vi "ENPID.vi"(2 "PID Settings":T1={"Gains"={"K(e)"=0.0, "Kp"=0.800000011920929, "Ki"=0.0, "Kd"=0.003000000026077032}, "Non-linear gain"={"Non-linear gain P"=enum."off", "Non-linear gain I"=enum."off", "Non-linear gain D"=enum."off"}, "D-Part variable"=enum."process variable", "Velocity estimate dy/dt"=enum."external", "Anti reset windup"=TRUE, "I-Part error band"=inf, "Output range"={"output high"=0.0, "output low"=0.0}}, 7 "r":dbl, 8 "Reset?":bool, 9 "y":dbl, 11 "dy/dt":dbl, 13 "dt (s)":dbl) -> (15 "u":dbl, 18 "u":cluster{"up":dbl, "ui":dbl, "ud":dbl, "u":dbl})   [LabVIEW 2019]
uses:
  PID_Settings.ctl
  Gains.ctl
  NonLinearGainParams.ctl
  NonLinearGain.ctl
  DPartVariable.ctl
  VelocityEstimate.ctl
  OutputRange.ctl
panel:
  # "Params"
  # "Input"
  # "Output"
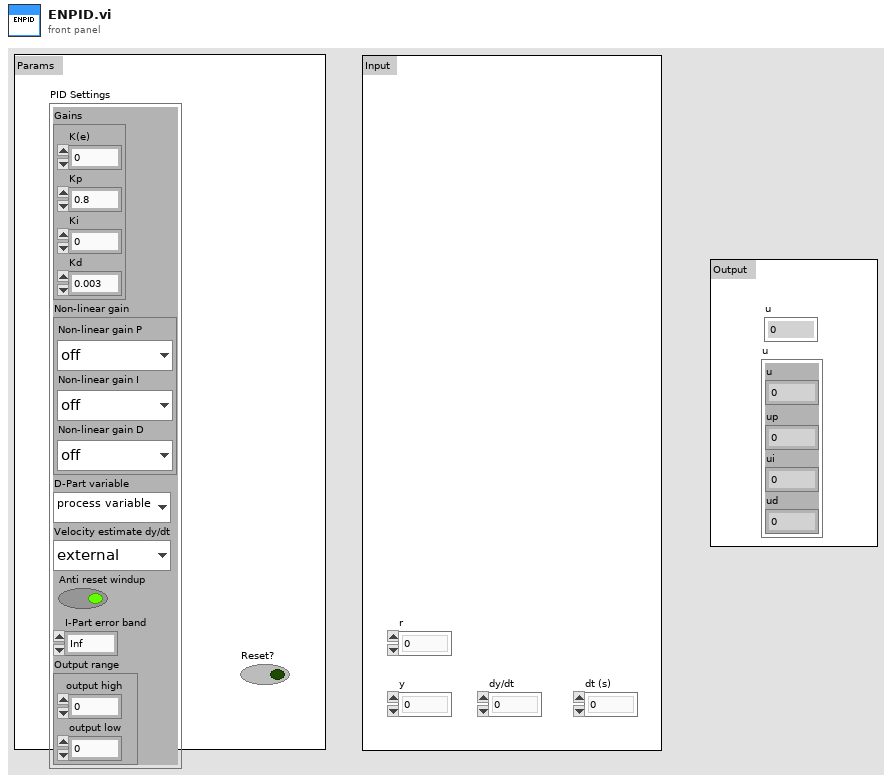
[diagram p1: front panel]
types:
  T1 = typedef "PID_Settings.ctl" = cluster{"Gains":T2, "Non-linear gain":T3, "D-Part variable":T5, "Velocity estimate dy/dt":T6, "Anti reset windup":bool, "I-Part error band":dbl, "Output range":T7}
  T2 = typedef "Gains.ctl" = cluster{"K(e)":dbl, "Kp":dbl, "Ki":dbl, "Kd":dbl}
  T3 = typedef "NonLinearGainParams.ctl" = cluster{"Non-linear gain P":T4, "Non-linear gain I":T4, "Non-linear gain D":T4}
  T4 = typedef "NonLinearGain.ctl" = enum16{"exponential", "quadratic", "off"}
  T5 = typedef "DPartVariable.ctl" = enum16{"error", "process variable"}
  T6 = typedef "VelocityEstimate.ctl" = enum16{"derivative", "external"}
  T7 = typedef "OutputRange.ctl" = cluster{"output high":dbl, "output low":dbl}
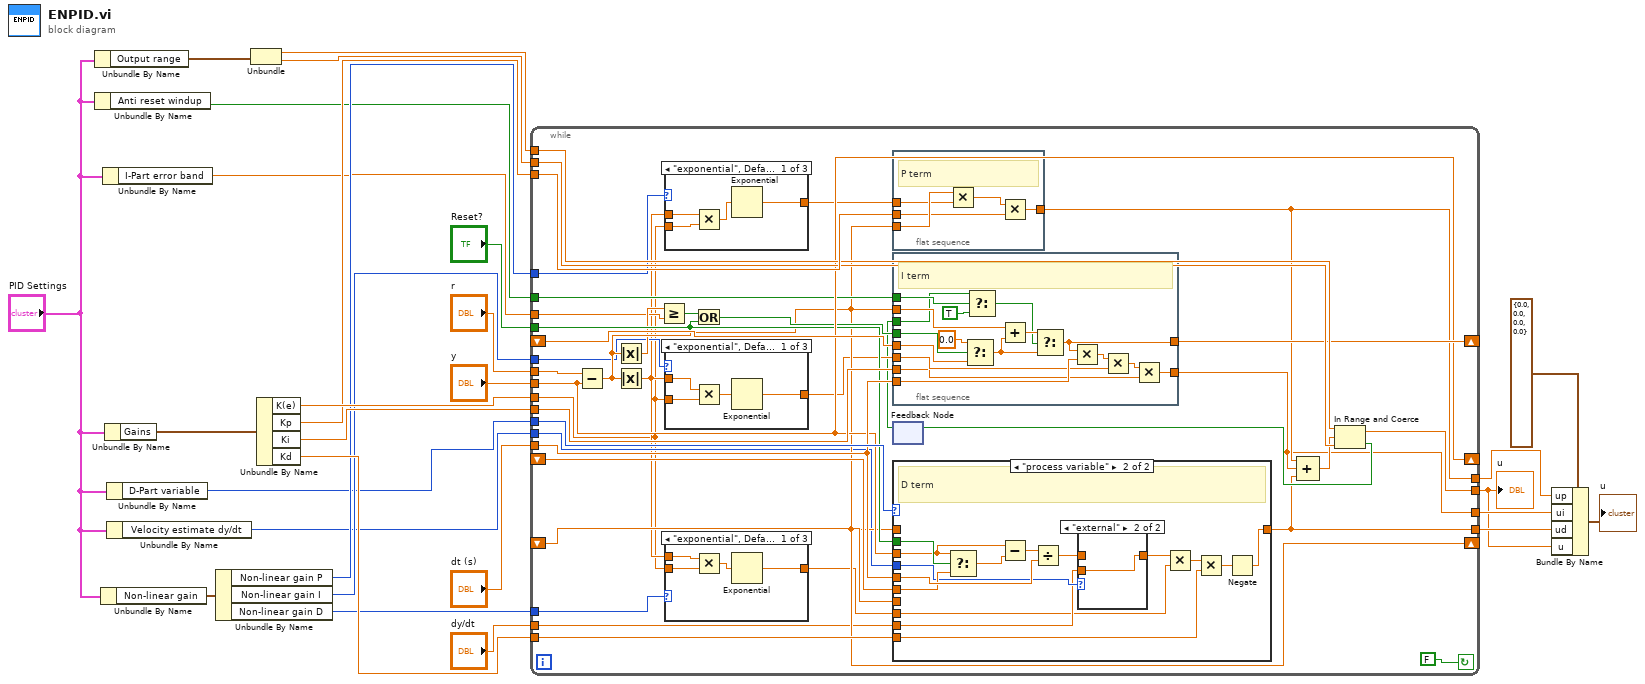
[diagram p0: block diagram]
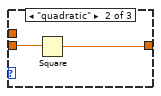
[diagram p2: hidden frame]
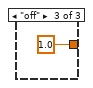
[diagram p3: hidden frame]
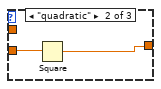
[diagram p4: hidden frame]
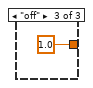
[diagram p5: hidden frame]
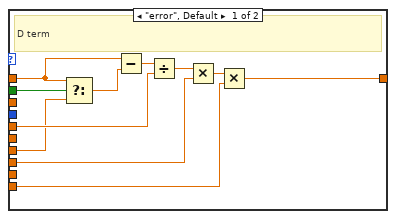
[diagram p6: hidden frame]
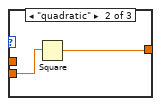
[diagram p8: hidden frame]
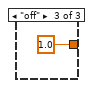
[diagram p9: hidden frame]
diagram:
  n1 = Unbundle By Name("PID Settings") -> ("Output range"=w2:T7)
  n2 = Unbundle By Name("PID Settings") -> ("Anti reset windup"=w7:bool)
  n3 = Unbundle By Name("PID Settings") -> ("Non-linear gain"=w8:T3)
  n4 = Unbundle By Name("PID Settings") -> ("I-Part error band"=w6:dbl)
  n5 = Unbundle By Name("PID Settings") -> ("Gains"=w9:T2)
  n6 = Unbundle By Name("PID Settings") -> ("D-Part variable"=w5:T5)
  n7 = Unbundle By Name("PID Settings") -> ("Velocity estimate dy/dt"=w4:T6)
  n8 = Unbundle By Name(w8) -> ("Non-linear gain P"=w10:T4, "Non-linear gain I"=w12:T4, "Non-linear gain D"=w11:T4)
  n9 = Unbundle(w2) -> ("output high"=w23:dbl, "output low"=w24:dbl)
  n10 = Unbundle By Name(w9) -> ("K(e)"=w28:dbl, "Kp"=w25:dbl, "Ki"=w20:dbl, "Kd"=w19:dbl)
  n11 = while {
    tunnel: w28 -> [w35]
    tunnel: "r" -> [w66]
    tunnel: "y" -> [w53]
    tunnel: w25 -> [w65]
    shift-right: [w42] -> _
    shift-left: _ -> [w50]
    tunnel: [w63] -> w1
    tunnel: w24 -> [w62]
    tunnel: w23 -> [w61]
    tunnel: "Reset?" -> [w45]
    tunnel: "dt (s)" -> [w55]
    tunnel: w20 -> [w56]
    shift-right: [w59] -> _
    shift-left: _ -> [w58]
    tunnel: w5 -> [w57]
    tunnel: w19 -> [w54]
    shift-right: [w53] -> _
    shift-left: _ -> [w52]
    tunnel: [w49] -> w18
    tunnel: [w48] -> w17
    tunnel: [w47] -> w16
    tunnel: w7 -> [w46]
    tunnel: w6 -> [w40]
    tunnel: "dy/dt" -> [w39]
    tunnel: w4 -> [w38]
    tunnel: w12 -> [w37]
    tunnel: w11 -> [w34]
    tunnel: w10 -> [w33]
    stop <- FALSE continue-if-true
    n12 = Subtract(x=w66, y=w53) -> (x-y=w42:dbl)
    n13 = Absolute Value(x=w42) -> (abs(x)=w41:dbl)
    n14 = Absolute Value(x=w42) -> (abs(x)=w36:dbl)
    n15 = Greater Or Equal?(x=w41, y=w40) -> (x >= y?=w43:bool)
    n16 = case shown="\"exponential\", Default" w33 {
      tunnel: w35 -> [w132 w136 _]
      tunnel: [w134 w135 1.0] -> w32
      tunnel: w36 -> [w131 _ _]
      frame "exponential", Default {
        n17 = Multiply(x=w131, y=w132) -> (x*y=w133:dbl)
        n18 = Exponential(1:w133) -> (0:w134:dbl)
      }
      frame "quadratic" {
        n19 = Square(x=w136) -> (x^2=w135:dbl)
      }
      frame "off" {
      }
    }
    n20 = case shown="\"exponential\", Default" w37 {
      tunnel: w35 -> [w75 w79 _]
      tunnel: [w77 w78 1.0] -> w30
      tunnel: w36 -> [w74 _ _]
      frame "exponential", Default {
        n21 = Multiply(x=w74, y=w75) -> (x*y=w76:dbl)
        n22 = Exponential(1:w76) -> (0:w77:dbl)
      }
      frame "quadratic" {
        n23 = Square(x=w79) -> (x^2=w78:dbl)
      }
      frame "off" {
      }
    }
    n24 = case shown="\"exponential\", Default" w34 {
      tunnel: w35 -> [w68 w72 _]
      tunnel: [w70 w71 1.0] -> w31
      tunnel: w36 -> [w67 _ _]
      frame "exponential", Default {
        n25 = Multiply(x=w67, y=w68) -> (x*y=w69:dbl)
        n26 = Exponential(1:w69) -> (0:w70:dbl)
      }
      frame "quadratic" {
        n27 = Square(x=w72) -> (x^2=w71:dbl)
      }
      frame "off" {
      }
    }
    n28 = Or(x=w43, y=w45) -> (x .or. y?=w44:bool)
    n29 = flat-sequence {
      tunnel: w42 -> [w130]
      tunnel: w32 -> [w126]
      tunnel: w65 -> [w128]
      tunnel: [w127] -> w49
      frame #0 {
        # "P term"
        n30 = Multiply(x=w130, y=w126) -> (x*y=w129:dbl)
        n31 = Multiply(x=w129, y=w128) -> (x*y=w127:dbl)
      }
    }
    n32 = flat-sequence {
      tunnel: w42 -> [w125]
      tunnel: w44 -> [w123]
      tunnel: w55 -> [w120]
      tunnel: w30 -> [w118]
      tunnel: w56 -> [w116]
      tunnel: [w115] -> w48
      tunnel: [w114] -> w59
      tunnel: w58 -> [w113]
      tunnel: w29 -> [w110]
      tunnel: w46 -> [w112]
      frame #0 {
        # "I term"
        n33 = Select(t=0.0, s=w123, f=w113) -> (s? t:f=w121:dbl)
        n34 = Select(t=w110, s=w112, f=TRUE) -> (s? t:f=w109:bool)
        n35 = Add(x=w125, y=w121) -> (x+y=w122:dbl)
        n36 = Select(t=w122, s=w109, f=w121) -> (s? t:f=w114:dbl)
        n37 = Multiply(x=w114, y=w120) -> (x*y=w119:dbl)
        n38 = Multiply(x=w119, y=w118) -> (x*y=w117:dbl)
        n39 = Multiply(x=w117, y=w116) -> (x*y=w115:dbl)
      }
    }
    n40 = feedback #1() -> (w29:bool)  [unwired: 1 in]
    n41 = case shown="\"process variable\"" w57 {
      tunnel: w42 -> [w83 _]
      tunnel: w50 -> [w84 _]
      tunnel: w55 -> [w90 w104]
      tunnel: w31 -> [w81 w92]
      tunnel: w54 -> [w87 w105]
      tunnel: [w86 w102] -> w47
      tunnel: w53 -> [_ w97]
      tunnel: w52 -> [_ w99]
      tunnel: w45 -> [w85 w100]
      tunnel: w39 -> [_ w95]
      tunnel: w38 -> [_ w96]
      frame "error", Default {
        # "D term"
        n42 = Select(t=w83, s=w85, f=w84) -> (s? t:f=w82:dbl)
        n43 = Subtract(x=w83, y=w82) -> (x-y=w91:dbl)
        n44 = Divide(x=w91, y=w90) -> (x/y=w89:dbl)
        n45 = Multiply(x=w89, y=w81) -> (x*y=w88:dbl)
        n46 = Multiply(x=w88, y=w87) -> (x*y=w86:dbl)
      }
      frame "process variable" {
        # "D term"
        n47 = Select(t=w97, s=w100, f=w99) -> (s? t:f=w98:dbl)
        n48 = Subtract(x=w97, y=w98) -> (x-y=w103:dbl)
        n49 = Divide(x=w103, y=w104) -> (x/y=w94:dbl)
        n50 = case shown="\"external\"" w96 {
          tunnel: w95 -> [_ w108]
          tunnel: [w107 w108] -> w93
          tunnel: w94 -> [w107 _]
          frame "derivative", Default {
          }
          frame "external" {
          }
        }
        n51 = Multiply(x=w93, y=w92) -> (x*y=w106:dbl)
        n52 = Multiply(x=w106, y=w105) -> (x*y=w101:dbl)
        n53 = Negate(x=w101) -> (-x=w102:dbl)
      }
    }
    n54 = Compound Arithmetic op=ADD(w49, w48, w47) -> (w60:dbl)
    n55 = In Range and Coerce(upper limit=w61, x=w60, lower limit=w62) -> (coerced(x)=w63:dbl, In Range?=w51:bool)
    n56 = feedback-in #1(w51) -> ()
  }
  "u" <- w1
  n57 = Bundle By Name(cluster=cluster{"up":dbl, "ui":dbl, "ud":dbl, "u":dbl} {"up"=0.0, "ui"=0.0, "ud"=0.0, "u"=0.0}, "up"=w18, "ui"=w17, "ud"=w16, "u"=w1) -> (→"u":cluster{"up":dbl, "ui":dbl, "ud":dbl, "u":dbl})
